vi "_UserDialog Choose ReadMe Params.vi"(0 "VI Default Path":path, 1 "LV <help> directory?":bool, 2 "Documentable VI Path":path, 7 "Info extracted from old HTML":T1={"_vi_name_"="", "_vi_description_text_"="", "_vi_controls_and_indicators_descriptions_"="", "_name_of_owning_library_"="", "_owning_library_html_"="", "_Packages_"="Base Package", "_Platforms_"="Windows", "_details_text_"="Put details here", "_example_screenshot_"="", "_example_vi_"="", "_path_to_example_file_"=path "", "IsDetailsON?"=FALSE, "IsOwningLibraryON?"=FALSE, "IsExamplesON?"=FALSE, "IsTableON?"=FALSE, "IsScrollableON?"=FALSE, "IsDetailedHelpLinkON?"=FALSE, "Table Objects array"=[], "Table Descriptions array"=[], "Table Links array"=[], "Start path location"=enum."VI folder"}, 11 "error in (no error)":errorcluster) -> (4 "HTML File Path":path, 8 "VI Info":T1={"_vi_name_"="", "_vi_description_text_"="", "_vi_controls_and_indicators_descriptions_"="", "_name_of_owning_library_"="", "_owning_library_html_"="", "_Packages_"="Base Package", "_Platforms_"="Windows", "_details_text_"="Put details here", "_example_screenshot_"="", "_example_vi_"="", "_path_to_example_file_"=path "", "IsDetailsON?"=FALSE, "IsOwningLibraryON?"=FALSE, "IsExamplesON?"=FALSE, "IsTableON?"=FALSE, "IsScrollableON?"=FALSE, "IsDetailedHelpLinkON?"=FALSE, "Table Objects array"=[], "Table Descriptions array"=[], "Table Links array"=[], "Start path location"=enum."VI folder"}, 14 "Cancelled by User?":bool, 15 "error out":errorcluster)   [LabVIEW 2012]
uses:
  _Controls and TypeDefs/UserDialogStates.ctl
  _Controls and TypeDefs/InfoFromOldHTML_cluster.ctl
  _Controls and TypeDefs/StartPathLocation_enum.ctl
  <vilib>/Platform/browser.llb/Open URL in Default Browser (string).vi
panel:
  in  "www.labicom.net":bool
  in  "Help Button":bool
  in  "Disclaimer":string="[Disclaimer text]"
  in  "IsDisclaimer? chkBox":bool=TRUE
  in  "Cancel Button":bool
  in  "GenerateReadme_btn":bool
  in  "Patents":string="[Patents text]"
  in  "Trademarks":string="[Trademarks text]"
  in  "Copyright":string="[Copyright text]"
  in  "Support CommunityForums":string=" [link to community forums or NI Community page and expected response time]"
  in  "SupportEmail":string="[Support email address and expected response time]"
  in  "SupportTelephone":string="[Telephone number and hours of operation]"
  in  "AppUpgrader":string="[Developer Name, Developer e-mail, Developer certification level (if any), Organization]"
  out "Product Version 8":string="[Version#]" caption="Product Version"
  in  "AppDeveloper":string="[Developer Name, Developer e-mail, Developer certification level (if any), Organization]"
  out "Product Short Name 12":string="[ProductShortName]" caption="Product Short Name"
  in  "IsDeveloper? chkBox":bool=TRUE
  in  "FixedIssues Table":string[][](table)=[["[#]", "[Summary Text]"], ["", ""], ["", ""]]
  out "Product Version 7":string="[Version#]" caption="Product Version"
  out "Product Short Name 11":string="[ProductShortName]" caption="Product Short Name"
  in  "NewFeatures Table":string[][](table)=[["[Feature 1]"], ["[Feature 2]"], [""]]
  out "Product Version 6":string="[Version#]" caption="Product Version"
  out "Product Short Name 10":string="[ProductShortName]" caption="Product Short Name"
  out "Product Version 5":string="[Version#]" caption="Product Version"
  out "Product Short Name 9":string="[ProductShortName]" caption="Product Short Name"
  in  "UpgradeIssuesDescription":string="[Description of known upgrade issue included recommended workaround.]"
  in  "Upgrade Issue Heading":string="[Upgrade Issue Heading]"
  out "Product Short Name 8":string="[ProductShortName]" caption="Product Short Name"
  in  "Device Support Table":string[][](table)=[["[Device]"], ["[Device]"], [""]]
  out "Product Short Name 7":string="[ProductShortName]" caption="Product Short Name"
  out "Product Short Name 6":string="[ProductShortName]" caption="Product Short Name"
  in  "NI Software Support Table":string[][](table)=[["LabVIEW", "8.5.x, 8.6.x, 2009 and later"], ["LabVIEW Real-Time Module", "8.5.x and later (including 2009 and later)"]]
  out "Product Version 4":string="[Version#]" caption="Product Version"
  out "Product Short Name 5":string="[ProductShortName]" caption="Product Short Name"
  in  "Additional OS remarks":string="[ProductName] [Version#] supports Phar Lap only with the LabVIEW Real-Time Module 8.5 and later.\nTo find and download an earlier version of [ProductName] [Version#] that supports other operating systems, refer to [link to older versions]."
  in  "Caution Text":string
  in  "OS Note":string="[Support for Windows Server 2003 R2 may require ...]"
  in  "OperatingSystems Table":string[][](table)=[["Windows 7 (32-bit and 64-bit)"], [""], [""], [""], [""]]
  out "Product Version 3":string="[Version#]" caption="Product Version"
  out "Product Short Name 4":string="[ProductShortName]" caption="Product Short Name"
  out "Product Short Name 3":string="[ProductShortName]" caption="Product Short Name"
  in  "SystemRequirements Table":string[][](table)=[["Development", "1 GB", "1 GHz or better"], ["Deployment", "256 MB", "600 MHz or better"]]
  in  "Installation Instructions":string[][](table)=[["[Step 1]"], ["[Step 2]"], [""], [""]]
  out "Product Short Name 2":string="[ProductShortName]" caption="Product Short Name"
  in  "IsCopyright? chkBox":bool=TRUE
  in  "IsPatents? chkBox":bool=TRUE
  in  "IsFixedIssues? chkBox":bool=TRUE
  in  "IsDeviceSupport? chkBox":bool=TRUE
  in  "IsTrademarks? chkBox":bool=TRUE
  in  "IsContactSupport? chkBox":bool=TRUE
  in  "IsNewFeatures? chkBox":bool=TRUE
  in  "IsUpgradeIssues? chkBox":bool=TRUE
  in  "IsSoftwareSupport? chkBox":bool=TRUE
  in  "IsSysRequirements? chkBox":bool=TRUE
  in  "IsInstallation? chkBox":bool=TRUE
  out "Product Version 2":string="[Version#]" caption="Product Version"
  in  "Product Short Name":string="[ProductShortName]"
  in  "Year":string="[Year]"
  in  "Month":string="[Month]"
  in  "Product Version":string="[Version#]"
  in  "Product Full Name":string="[ProductFullName]"
  in  "Next_btn":bool
  in  "UserDialogSteps":T3=enum."Choose parameters"
  # "Readme"
  # "Thank you for using"
  # ", version"
  # "."
  # "The readme contains the following main sections:"
  # "Installation (if applicable)"
  # "."
  # "This section documents installation instructions for"
  # "New line here corresponds to new item in the list in HTML"
  # "System Requirements (if applicable)"
  # "Software Support in"
  # "(if applicable)"
  # "Operating System Support"
  # ":"
  # "The following operating systems are supported in"
  # "Step 2/2:\nConfigure VI Documentation Layout"
  # "Note"
  # "Additional layout elements for LabVIEW help"
  # "This icon denotes a note, which alerts you\nto important information. You can add it\nby placing <_note_> into your text."
  # "Caution: place <_caution_> into your text"
  # "Caution"
  # "Note: place <_note_> into your text"
  # "This icon denotes a caution, which \nadvises you of precautions to take to \navoid injury, data loss, or a system crash.\nYou can add it by placing <_caution_>\ninto your text."
  # "Mandatory Fields"
  # "Tip: place <_tip_> into your text"
  # "Windows"
  # "Platform: enclose platform name between\n<_platform_> and </_platform_> tags"
  # "Text in blue color denotes a specific \nplatform and indicates that the text \nfollowing it applies only to that platform.\nYou can add it enclosing platform name\nbetween <_platform_> and </_platform_>\ntags (e.g.: <_platform_>MacOS X</_platform_>)."
  # "NI Application Software Support"
  # "The following table lists the NI application software versions supported by"
  # "bold"
  # "Text in bold: enclose such text between\n<B> and </B> tags"
  # ":"
  # "Attention!"
  # "Caution Text: enclose such text between \n<_caution_text_> and </_caution_text_> tags"
  # "Bold text denotes items that you must \nselect or click on in the software, such as \nmenu items and dialog box options. \nBold text also denotes parameter names, \nemphasis, or an introduction to a key \nconcept. You can emphasize such text by \nenclosing in between <B> and </B> tags."
  # "vigods.com"
  # "Link: place relative path in place of '_path_' and\ntext in place of '_text_' and insert resulting string\nwherever you need: \n<a href=\"_path_\">_text_</a>"
  # "monospace"
  # "Monospace: enclose such text between\n<_monospace_> and </_monospace_> tags"
  # "Device Support in"
  # "(if applicable)"
  # "The following lists detail the devices supported in"
  # "."
  # "Upgrade and Compatibility Issues"
  # "(if applicable)"
  # "This section covers changes in"
  # "functionality."
  # "New Features Added in"
  # "(if applicable)"
  # ":"
  # "The following features were added in"
  # "Fixed Issues"
  # "(if applicable)"
  # "The following issues were fixed in"
  # "Developer(s) of"
  # "(if applicable)"
  # "This application was developed by"
  # "Last upgrade of this application (to the version"
  # ") was made by"
  # "Contact Support"
  # "(if applicable)"
  # "You can contact our support staff by one of the following:"
  # "Telephone:"
  # "Email:"
  # "Community Forums:"
  # "Copyright"
  # "(if applicable)"
  # "Trademarks"
  # "(if applicable)"
  # "Patents"
  # "(if applicable)"
  # "Disclaimer"
  # "(if applicable)"
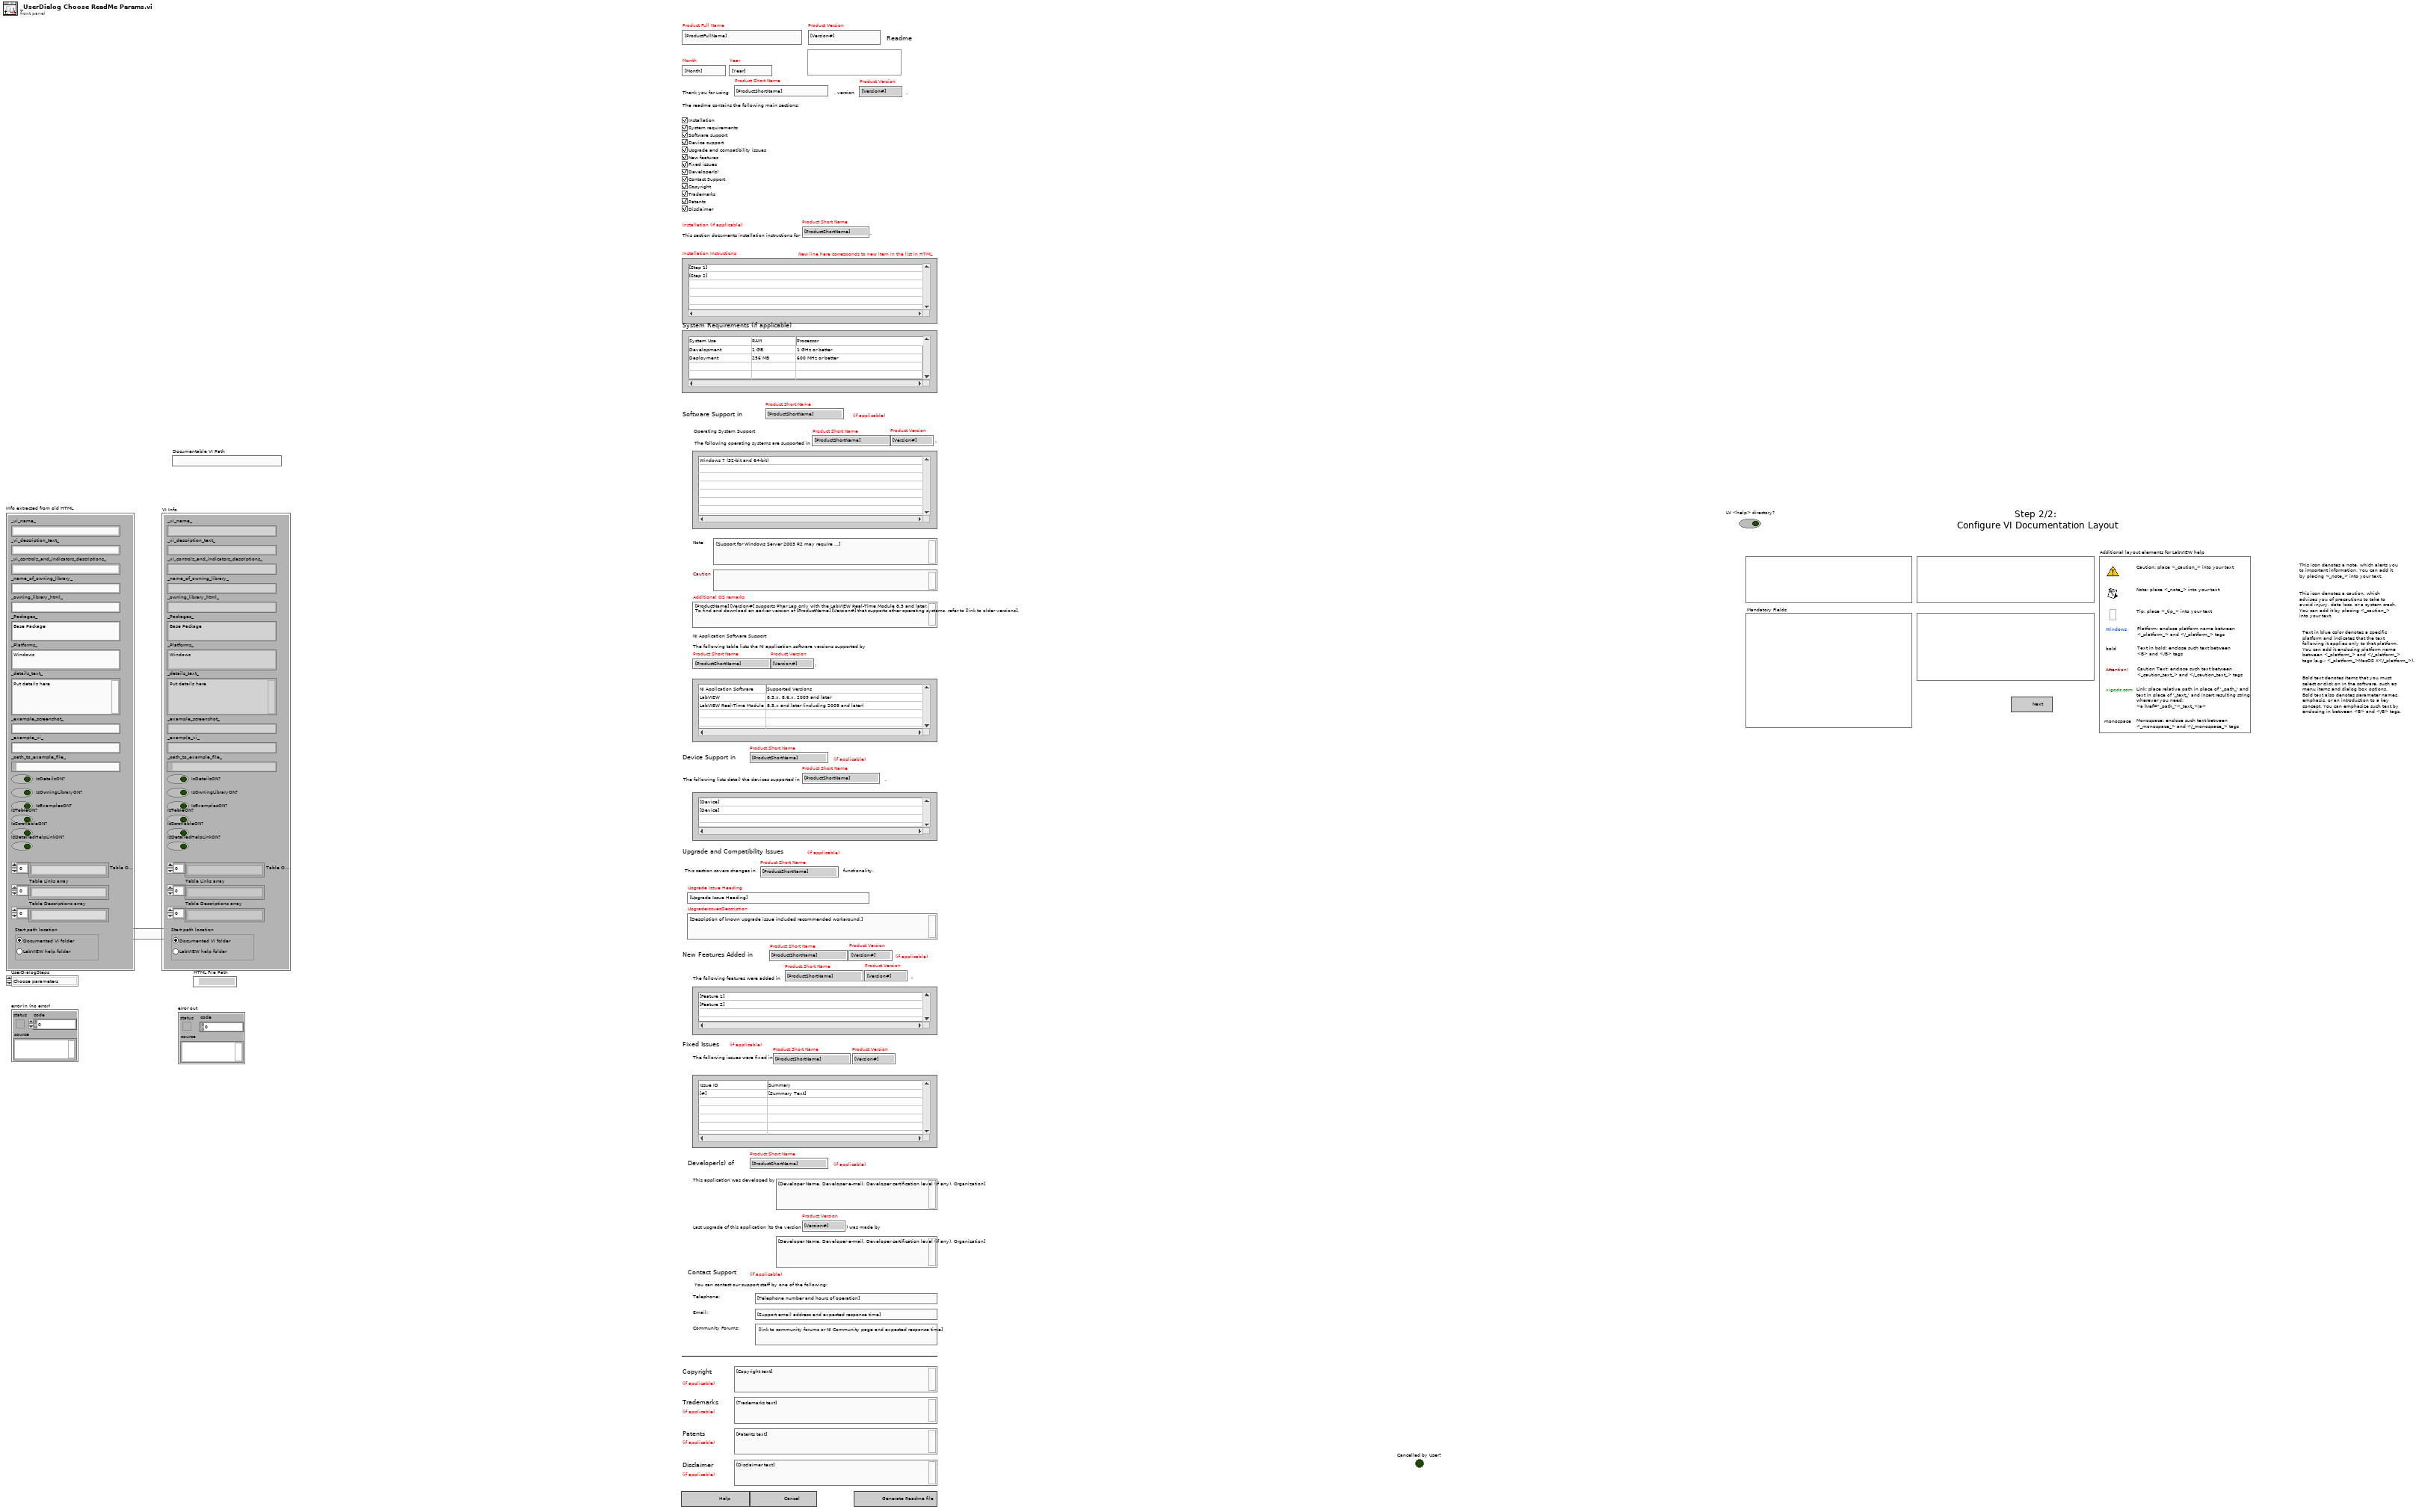
[diagram p1: front panel]
types:
  T1 = typedef "InfoFromOldHTML_cluster.ctl" = cluster{"_vi_name_":string, "_vi_description_text_":string, "_vi_controls_and_indicators_descriptions_":string, "_name_of_owning_library_":string, "_owning_library_html_":string, "_Packages_":string, "_Platforms_":string, "_details_text_":string, "_example_screenshot_":string, "_example_vi_":string, "_path_to_example_file_":path, "IsDetailsON?":bool, "IsOwningLibraryON?":bool, "IsExamplesON?":bool, "IsTableON?":bool, "IsScrollableON?":bool, "IsDetailedHelpLinkON?":bool, "Table Objects array":string[], "Table Descriptions array":string[], "Table Links array":string[], "Start path location":T2}
  T2 = typedef "StartPathLocation_enum.ctl" = enum32{"VI folder", "Help folder"}
  T3 = typedef "UserDialogStates.ctl" = enum16{"Overview", "Known Issues", "Choose parameters", "Update", "Choose HTML file path", "Choose Images directory path", "Decide if there is Context Help", "Choose help hierarchy", "Generate HTML", "Installation", "System Requirements", "Software Support", "Device Support", "Upgrade Issues", "New Features", "Fixed Issues", "Developer", "Contact Support", "Copyright", "Trademarks", "Patents", "Disclaimer", "Save", "Shutdown"}
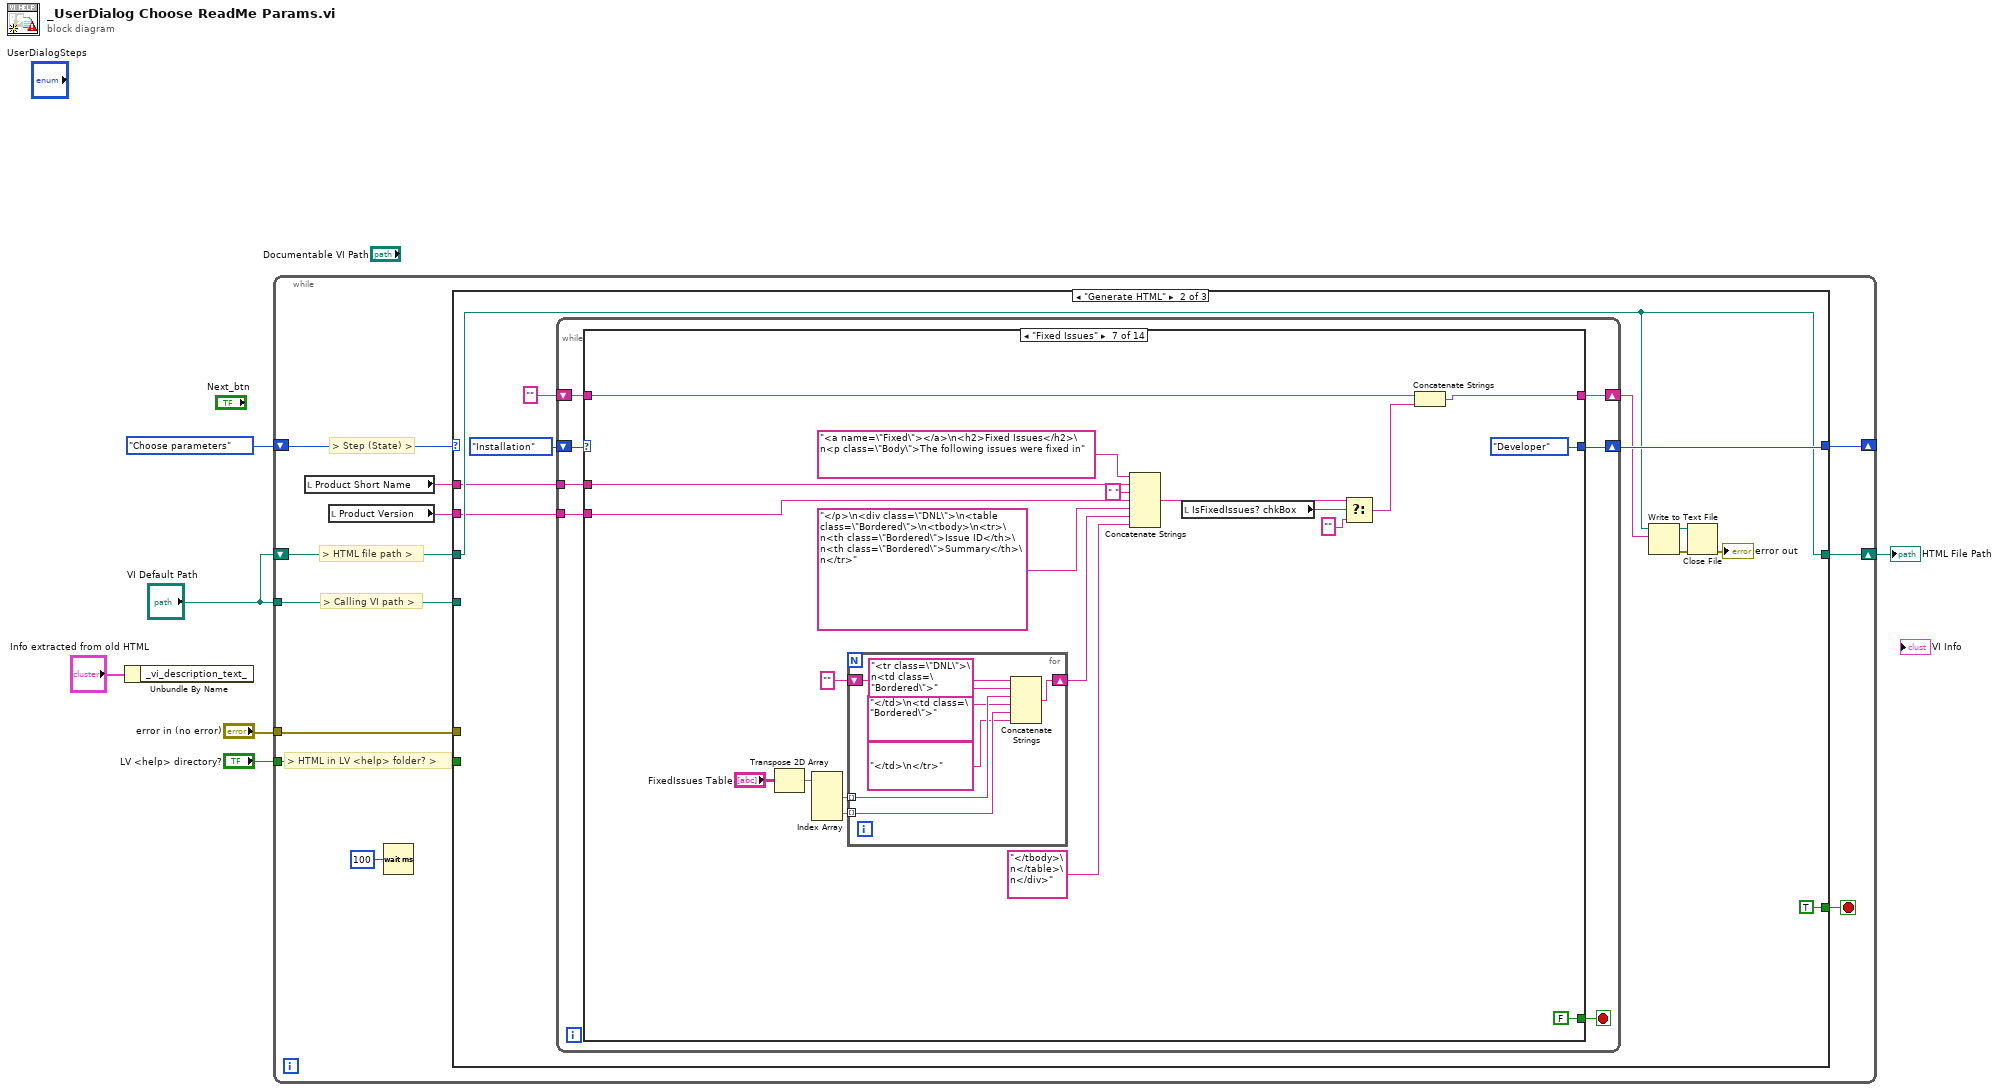
[diagram p0: block diagram]
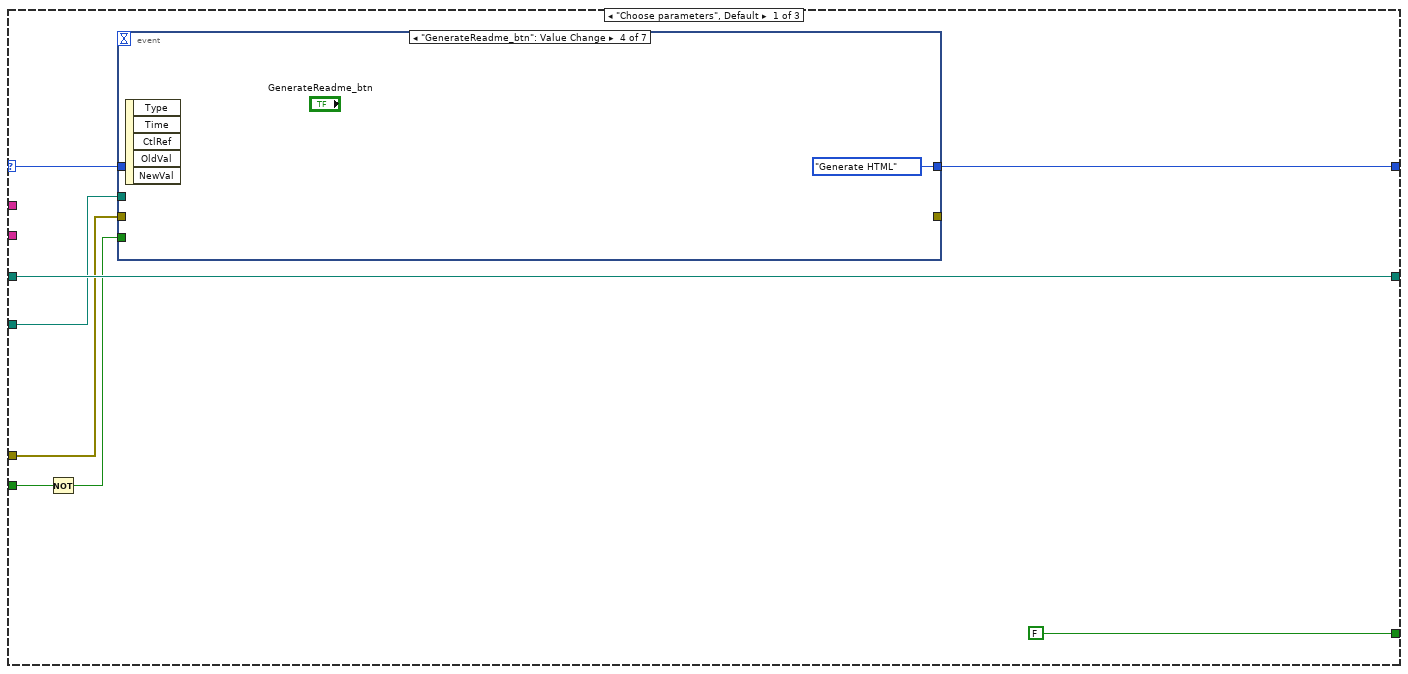
[diagram p2: hidden frame]
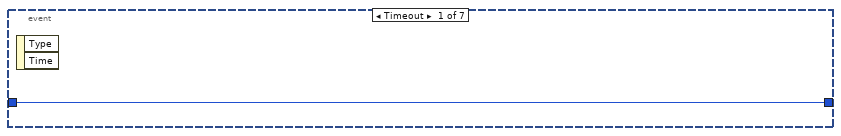
[diagram p3: hidden frame]
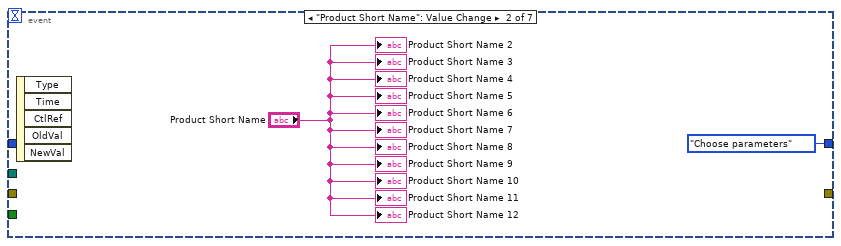
[diagram p4: hidden frame]
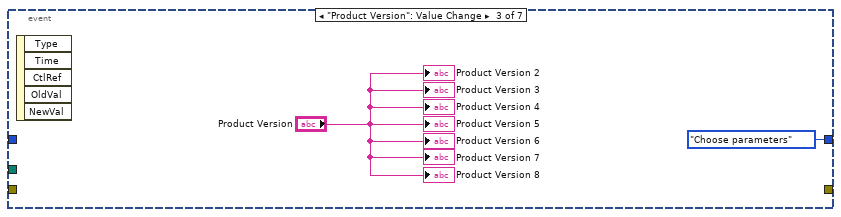
[diagram p5: hidden frame]
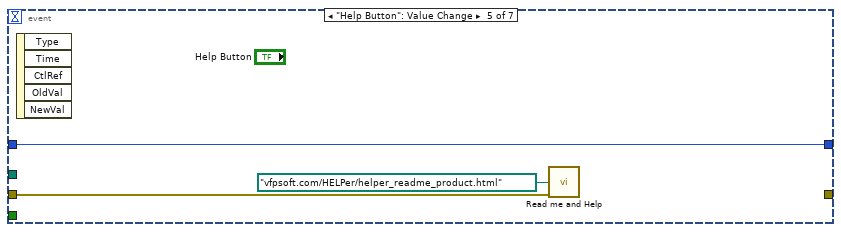
[diagram p6: hidden frame]
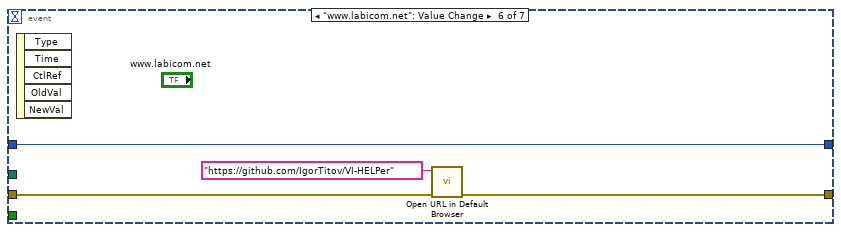
[diagram p7: hidden frame]
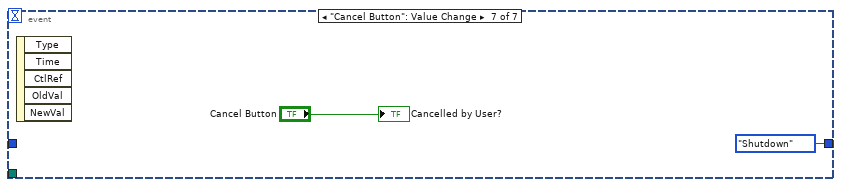
[diagram p8: hidden frame]
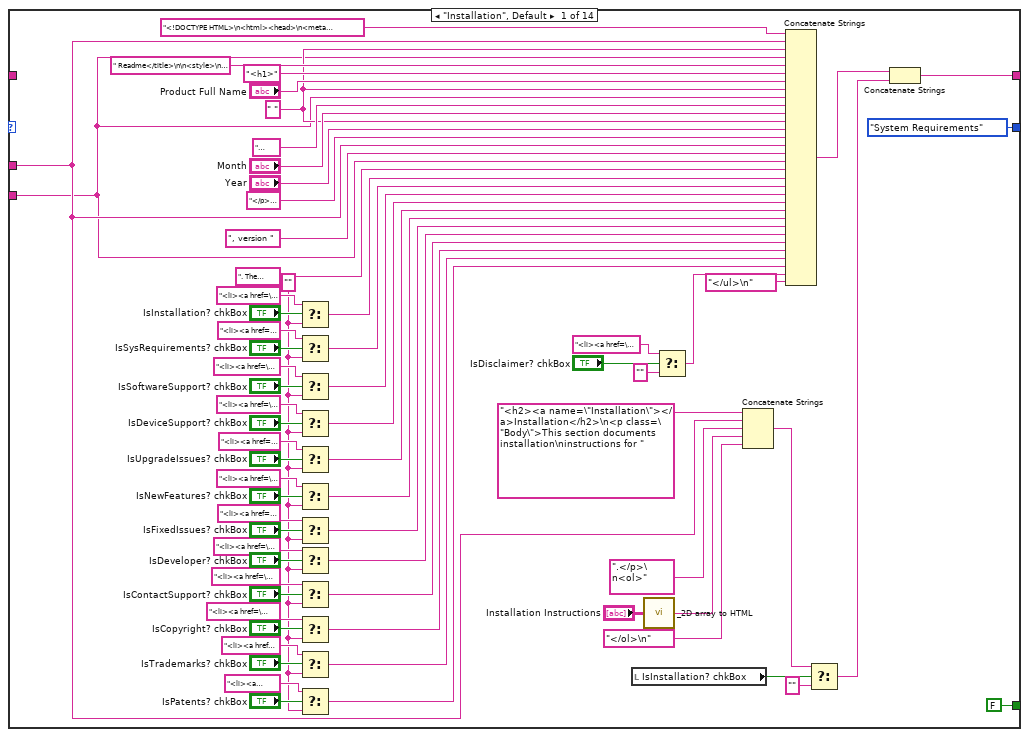
[diagram p9: hidden frame]
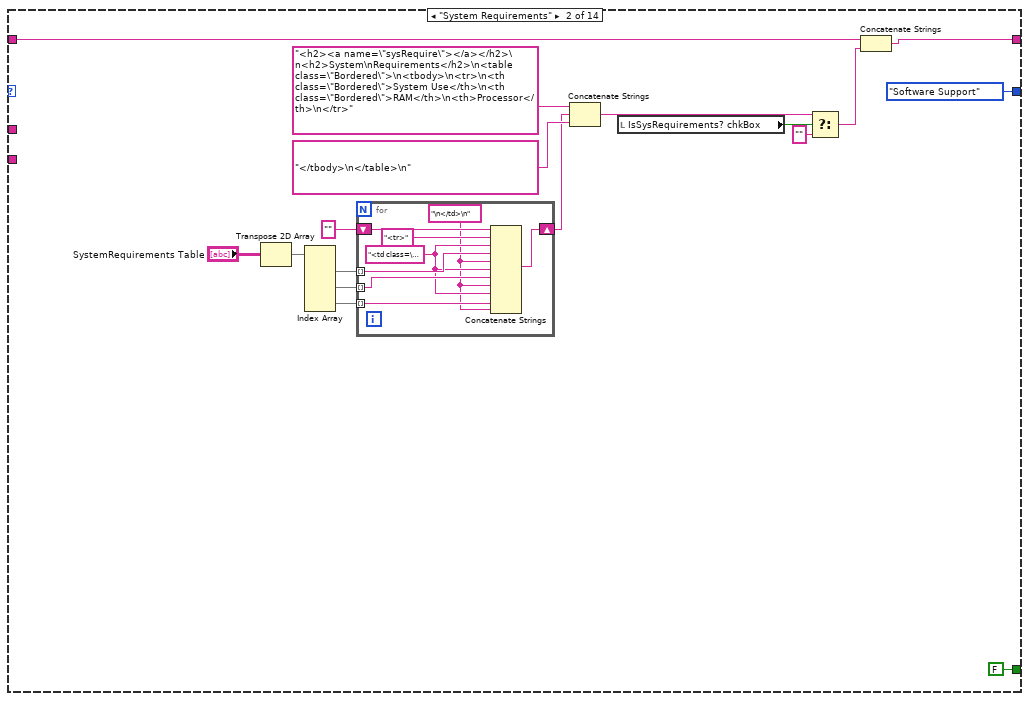
[diagram p10: hidden frame]
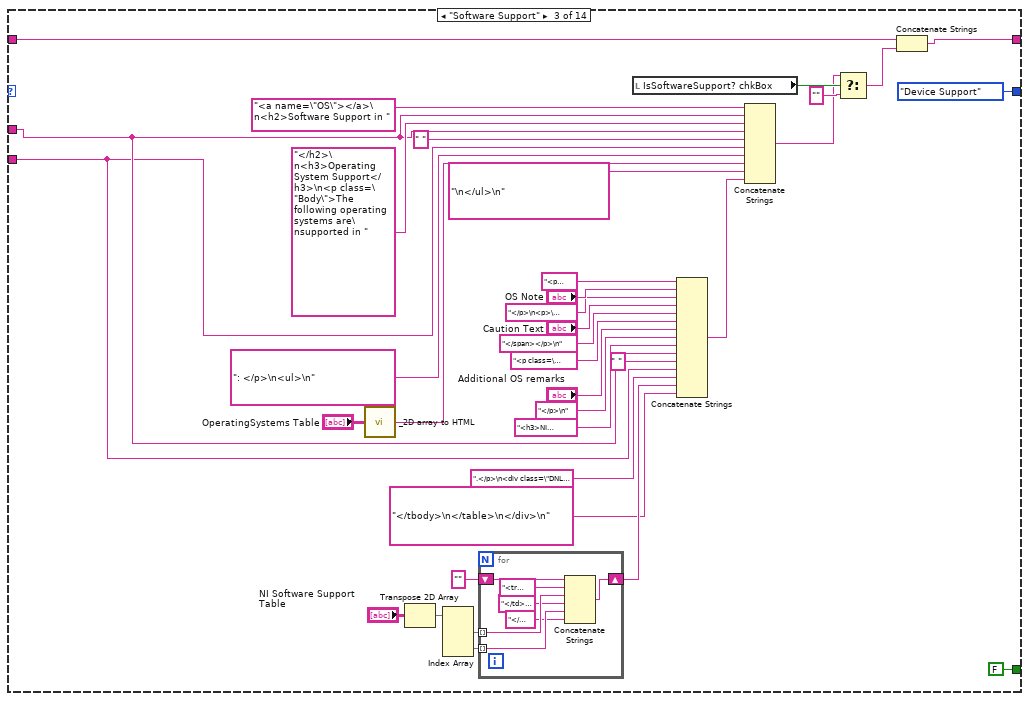
[diagram p11: hidden frame]
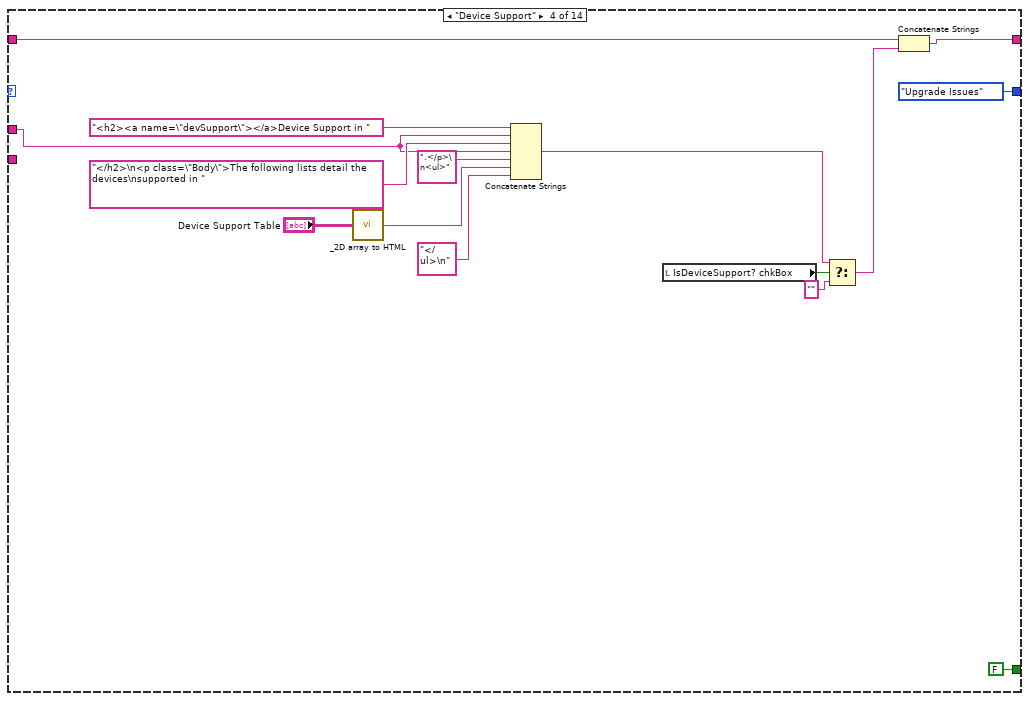
[diagram p12: hidden frame]
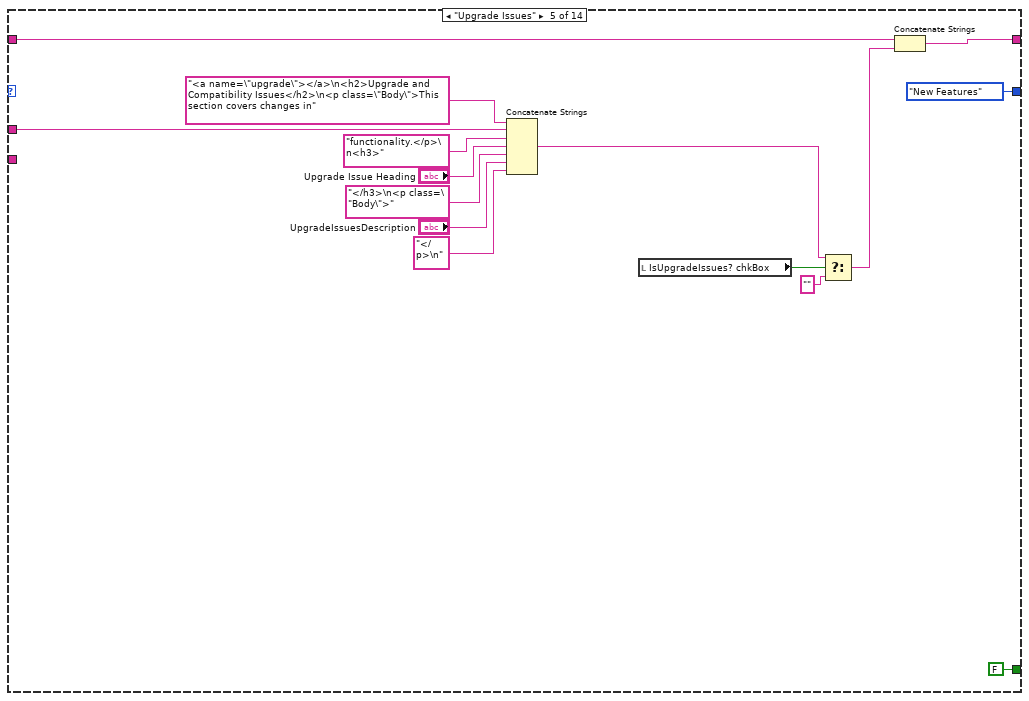
[diagram p13: hidden frame]
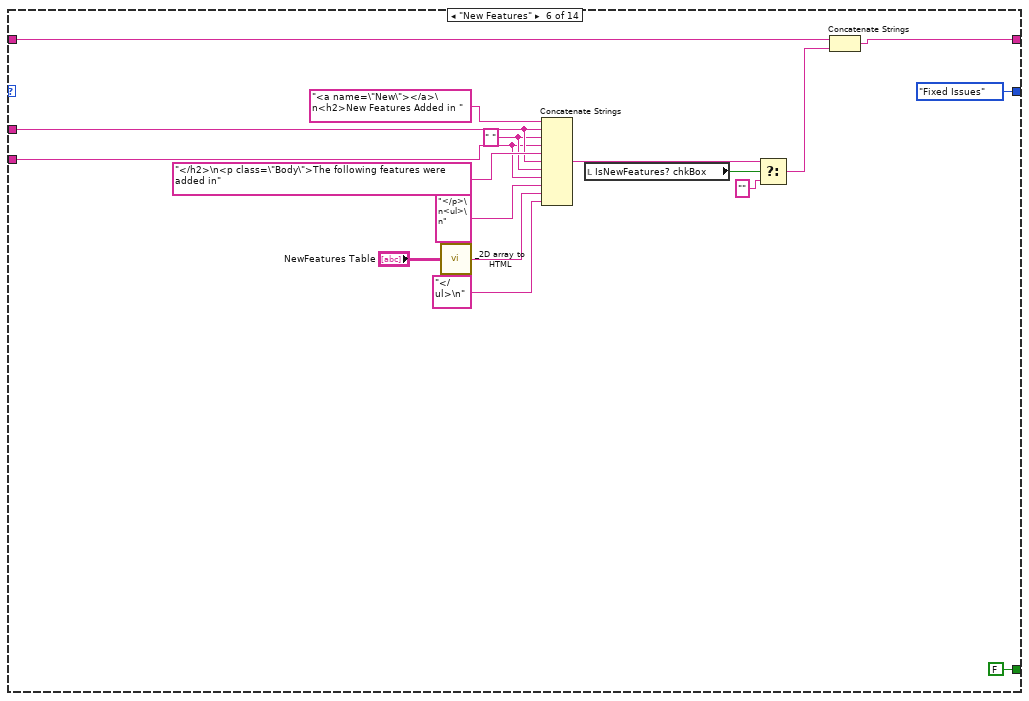
[diagram p14: hidden frame]
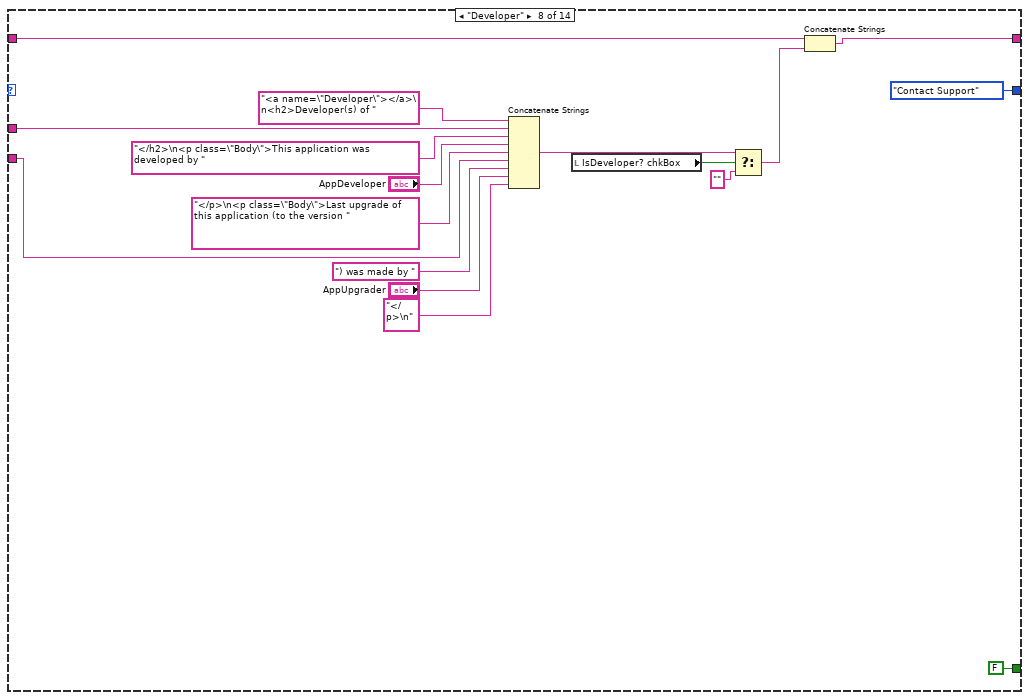
[diagram p15: hidden frame]
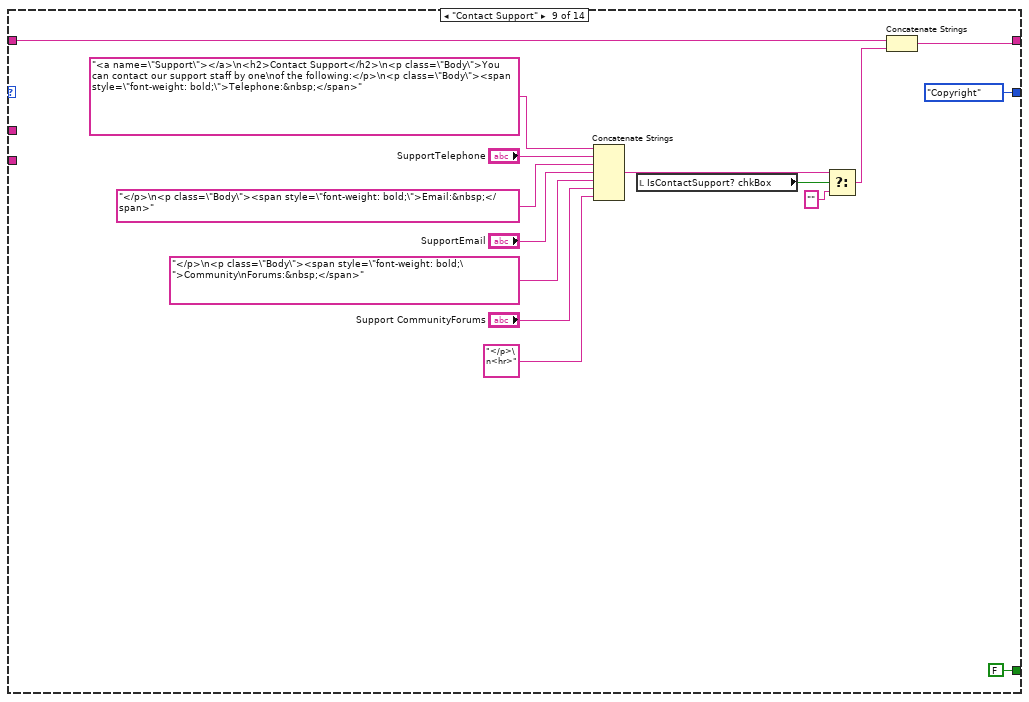
[diagram p16: hidden frame]
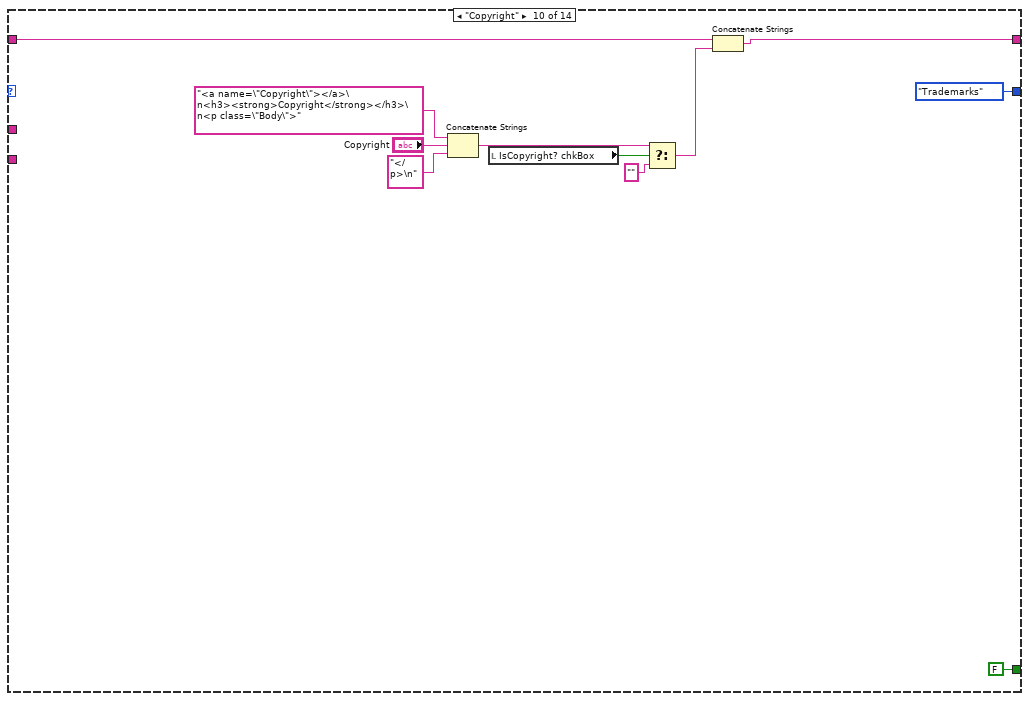
[diagram p17: hidden frame]
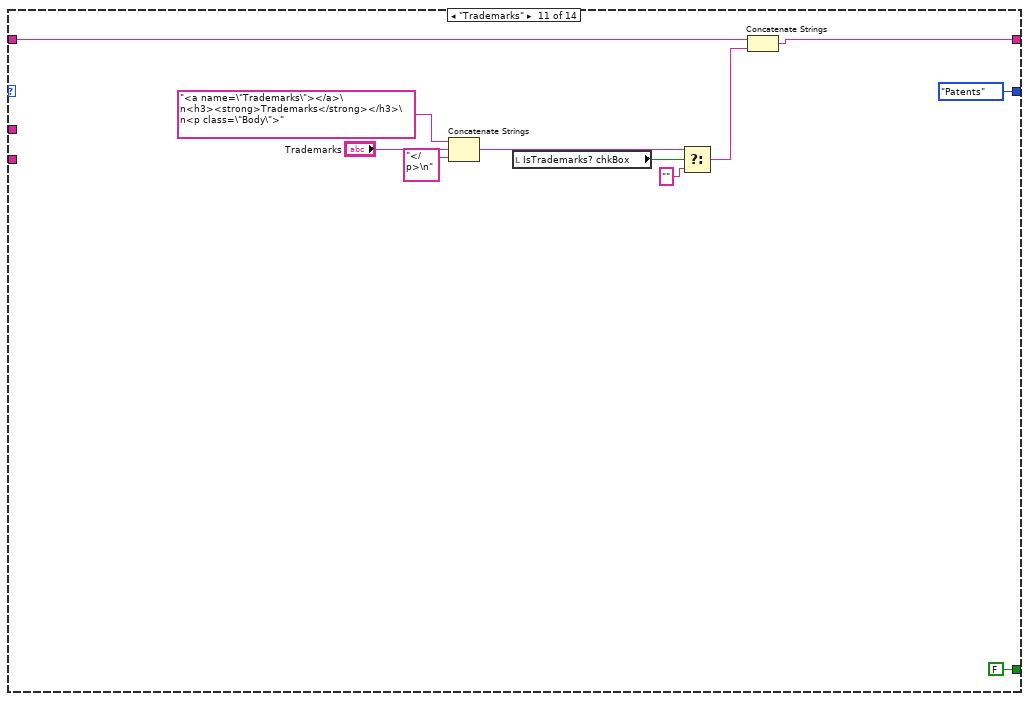
[diagram p18: hidden frame]
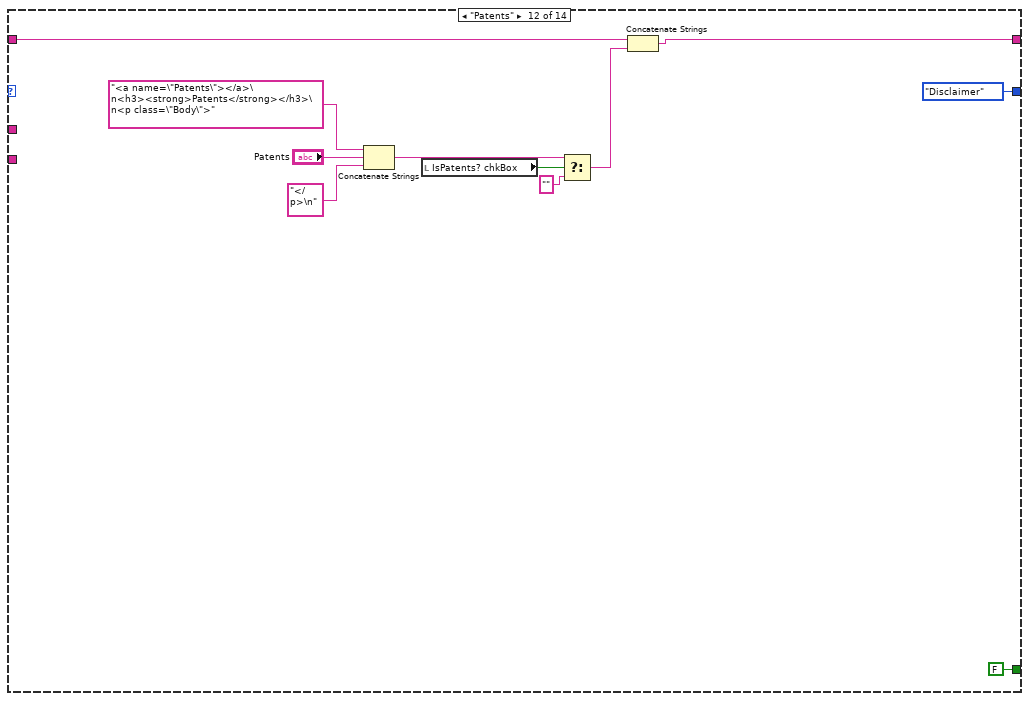
[diagram p19: hidden frame]
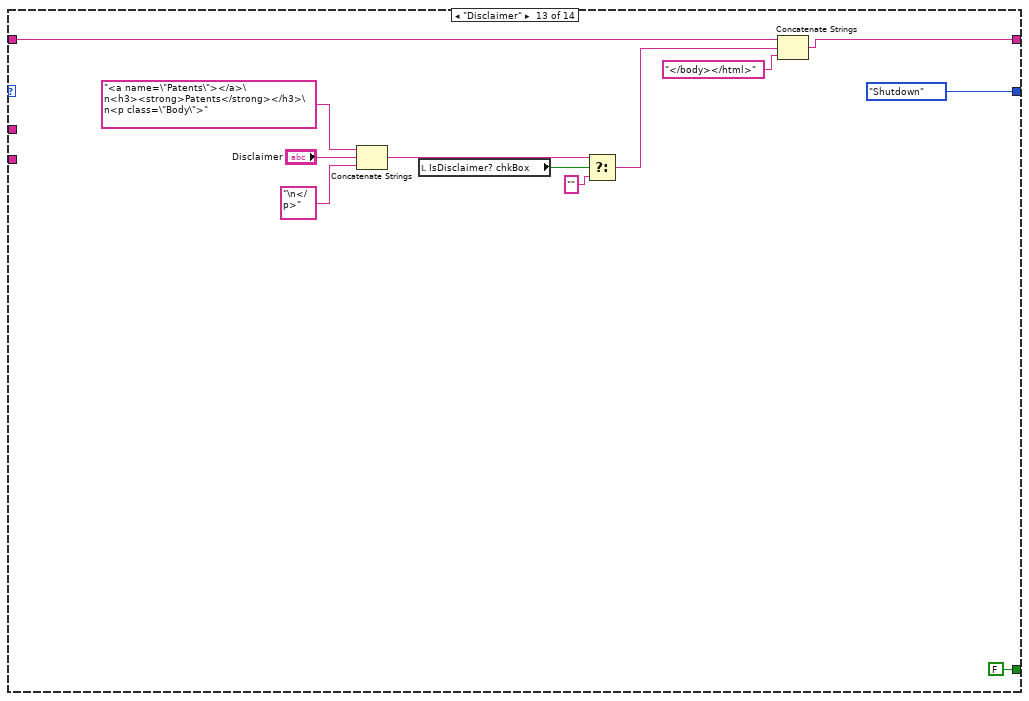
[diagram p20: hidden frame]
diagram:
  n1 = Unbundle By Name("Info extracted from old HTML") -> ()  [unwired: 1 out]
  n2 = while {
    shift-right: [w14] -> _
    shift-left: UserDialogStates."Choose parameters" ("UserDialogSteps") -> [w15]
    tunnel: "VI Default Path" -> [w13]
    shift-right: [w12] -> w3
    shift-left: "VI Default Path" -> [w11]
    tunnel: "LV <help> directory?" -> [w10]
    tunnel: "error in (no error)" -> [w9]
    stop <- w17 stop-if-true
    # "> HTML in LV <help> folder? >"
    # "> Step (State) >"
    # "> Calling VI path >"
    # "> HTML file path >"
    n3 = local read "Product Short Name"() -> (w8:string)
    n4 = local read "Product Version"() -> (w7:string)
    n5 = Wait (ms)(milliseconds to wait=u32 100) -> ()  [unwired: 1 out]
    n6 = case shown="\"Generate HTML\"" w15 {
      selector: w15 -> [w24 _ _]
      tunnel: [FALSE TRUE TRUE] -> w17
      tunnel: [w23 w49 UserDialogStates."Shutdown" ("UserDialogSteps")] -> w14
      tunnel: w13 -> [w20 _ _]
      tunnel: [w22 w47 w350] -> w12
      tunnel: w11 -> [w22 w47 w350]
      tunnel: w10 -> [w21 _ _]
      tunnel: w9 -> [w18 _ _]
      tunnel: w8 -> [_ w42 _]
      tunnel: w7 -> [_ w41 _]
      frame "Choose parameters", Default {
        n7 = Not(x=w21) -> (.not. x?=w19:bool)
        n8 = event shown="[3] \"GenerateReadme_btn\": Value Change" {
          selector: _ -> [_ _ _ _ _ _ _]
          dyn-events: _ -> [_ _ _ _ _ _ _]
          timeout: _ -> [_ _ _ _ _ _ _]
          tunnel: w24 -> [w26 _ _ _ w32 w38 _]
          tunnel: [w26 UserDialogStates."Choose parameters" ("UserDialogSteps") UserDialogStates."Choose parameters" ("UserDialogSteps") UserDialogStates."Generate HTML" ("UserDialogSteps") w32 w38 UserDialogStates."Shutdown" ("UserDialogSteps")] -> w23
          tunnel: w20 -> [_ _ _ _ _ _ _]
          tunnel: w19 -> [_ _ _ _ _ _ _]
          tunnel: w18 -> [_ _ _ _ w33 w36 _]
          tunnel: [_ _ _ _ _ w35 _] -> _
          event Timeout {
            n9 = event-data() -> ()  [unwired: 1 in, 2 out]
          }
          event "Product Short Name": Value Change {
            n10 = event-data() -> ()  [unwired: 1 in, 5 out]
            "Product Short Name 2" <- "Product Short Name"
            "Product Short Name 9" <- "Product Short Name"
            "Product Short Name 3" <- "Product Short Name"
            "Product Short Name 4" <- "Product Short Name"
            "Product Short Name 5" <- "Product Short Name"
            "Product Short Name 6" <- "Product Short Name"
            "Product Short Name 7" <- "Product Short Name"
            "Product Short Name 8" <- "Product Short Name"
            "Product Short Name 10" <- "Product Short Name"
            "Product Short Name 11" <- "Product Short Name"
            "Product Short Name 12" <- "Product Short Name"
          }
          event "Product Version": Value Change {
            n11 = event-data() -> ()  [unwired: 1 in, 5 out]
            "Product Version 2" <- "Product Version"
            "Product Version 3" <- "Product Version"
            "Product Version 4" <- "Product Version"
            "Product Version 5" <- "Product Version"
            "Product Version 6" <- "Product Version"
            "Product Version 7" <- "Product Version"
            "Product Version 8" <- "Product Version"
          }
          event "GenerateReadme_btn": Value Change {
            n12 = event-data() -> ()  [unwired: 1 in, 5 out]
          }
          event "Help Button": Value Change {
            n13 = event-data() -> ()  [unwired: 1 in, 5 out]
            n14 = call "Read me and Help.vi"("path"=path "vfpsoft.com/HELPer/helper_readme_product.html", "error in"=w33) -> ()  [unwired: 13 in, 1 out]
          }
          event "www.labicom.net": Value Change {
            n15 = event-data() -> ()  [unwired: 1 in, 5 out]
            n16 = call-poly <vilib>:"Open URL in Default Browser.vi"("error in (no error)"=w36, "URL"="https://github.com/IgorTitov/VI-HELPer") -> ("error out"=w35:errorcluster)  [unwired: 4 in, 1 out]
          }
          event "Cancel Button": Value Change {
            n17 = event-data() -> ()  [unwired: 1 in, 5 out]
            "Cancelled by User?" <- "Cancel Button"
          }
        }
      }
      frame "Generate HTML" {
        n18 = while {
          shift-right: [w57] -> w49
          shift-left: UserDialogStates."Installation" ("UserDialogSteps") -> [w58]
          shift-right: [w55] -> w46
          shift-left: "" -> [w56]
          tunnel: w42 -> [w53]
          tunnel: w41 -> [w52]
          stop <- w54 stop-if-true
          n19 = case shown="\"Fixed Issues\"" w58 {
            tunnel: [UserDialogStates."System Requirements" ("UserDialogSteps") UserDialogStates."Software Support" ("UserDialogSteps") UserDialogStates."Device Support" ("UserDialogSteps") UserDialogStates."Upgrade Issues" ("UserDialogSteps") UserDialogStates."New Features" ("UserDialogSteps") UserDialogStates."Fixed Issues" ("UserDialogSteps") UserDialogStates."Developer" ("UserDialogSteps") UserDialogStates."Contact Support" ("UserDialogSteps") UserDialogStates."Copyright" ("UserDialogSteps") UserDialogStates."Trademarks" ("UserDialogSteps") UserDialogStates."Patents" ("UserDialogSteps") UserDialogStates."Disclaimer" ("UserDialogSteps") UserDialogStates."Shutdown" ("UserDialogSteps") UserDialogStates."Shutdown" ("UserDialogSteps")] -> w57
            tunnel: w56 -> [_ w142 w176 w207 w219 w237 w257 w282 w296 w307 w318 w329 w340 w346]
            tunnel: [w80 w141 w175 w206 w220 w238 w256 w281 w295 w306 w317 w328 w343 w346] -> w55
            tunnel: [FALSE FALSE FALSE FALSE FALSE FALSE FALSE FALSE FALSE FALSE FALSE FALSE FALSE TRUE] -> w54
            tunnel: w53 -> [w60 _ w153 w195 w215 w234 w252 w276 _ _ _ _ _ _]
            tunnel: w52 -> [w59 _ w152 _ _ w232 w250 w272 _ _ _ _ _ _]
            frame "Installation", Default {
              w83 = ""
              w61 = " " ("string")
              n20 = Select(t="<li><a href=\"#Installation\">Installation</a></li>\n", s="IsInstallation? chkBox", f=w83) -> (s? t:f=w116:string)
              n21 = Select(t="<li><a href=\"#sysRequire\">System requirements</a></li>\n", s="IsSysRequirements? chkBox", f=w83) -> (s? t:f=w113:string)
              n22 = Select(t="<li><a href=\"#OS\">Software support</a></li>\n", s="IsSoftwareSupport? chkBox", f=w83) -> (s? t:f=w110:string)
              n23 = Select(t="<li><a href=\"#devSupport\">Device support</a></li>\n", s="IsDeviceSupport? chkBox", f=w83) -> (s? t:f=w108:string)
              n24 = Select(t="<li><a href=\"#upgrade\">Upgrade and compatibility issues</a></li>\n", s="IsUpgradeIssues? chkBox", f=w83) -> (s? t:f=w104:string)
              n25 = Select(t="<li><a href=\"#New\">New features</a></li>\n", s="IsNewFeatures? chkBox", f=w83) -> (s? t:f=w102:string)
              n26 = Select(t="<li><a href=\"#Fixed\">Fixed issues</a></li>\n", s="IsFixedIssues? chkBox", f=w83) -> (s? t:f=w99:string)
              n27 = Select(t="<li><a href=\"#Developer\">Developer(s)</a></li>", s="IsDeveloper? chkBox", f=w83) -> (s? t:f=w96:string)
              n28 = Select(t="<li><a href=\"#Support\">Contact Support</a></li>\n", s="IsContactSupport? chkBox", f=w83) -> (s? t:f=w93:string)
              n29 = Select(t="<li><a href=\"#Copyright\">Copyright</a></li>\n", s="IsCopyright? chkBox", f=w83) -> (s? t:f=w89:string)
              n30 = Select(t="<li><a href=\"#Trademarks\">Trademarks</a></li>\n", s="IsTrademarks? chkBox", f=w83) -> (s? t:f=w82:string)
              n31 = Select(t="<li><a href=\"#Patents\">Patents</a></li>\n", s="IsPatents? chkBox", f=w83) -> (s? t:f=w81:string)
              n32 = local read "IsInstallation? chkBox"() -> (w77:bool)
              n33 = call "_2D array to HTML.vi"("Table (2D Array)"="Installation Instructions") -> ("HTML Code"=w73:string)  [unwired: 14 in]
              n34 = Select(t="<li><a href=\"#Disclaimer\">Disclaimer</a></li>\n", s="IsDisclaimer? chkBox", f="") -> (s? t:f=w67:string)
              n35 = Concatenate Strings("<h2><a name=\"Installation\"></a>Installation</h2>\n<p class=\"Body\">This section documents installation\ninstructions for " ("string"), w60, ".</p>\n<ol>" ("string"), w73, "</ol>\n" ("string")) -> (w71:string)
              n36 = Concatenate Strings("<!DOCTYPE HTML>\n<html><head>\n<meta http-equiv=\"Content-Type\" content=\"text/html; charset=ISO-8859-1\">\n<META NAME=\"GENERATOR\" CONTENT=\"HELPer - VI Documentation Toolkit from https://github.com/IgorTitov/VI-HELPer\">\n<script>\nfunction Link(URL)\n{\nwindow.location = URL;\n}\n</script>\n<meta http-equiv=\"Content-Type\" content=\"text/html; charset=ISO-8859-1\"><title>", w60, w61, w59, " Readme</title>\n\n<style>\n/***************************************************/\n/* MINIMAL STYLES */\n/* The following section defines styles that every HTML Help project should\nneed. */\n/* The default style of P is red to alert you that you need to apply a style\nclass, such as Body. */\nP { margin-top:6.00pt; margin-bottom:6.00pt; font-family:Verdana; font-size:8pt;\ncolor: #FF0000; }\nBR { font-size:4.00pt; }\n/* Use H1 for all topic headings. */\nH1 { margin-top:3.00pt; margin-bottom:3.00pt; font-family:Verdana;\nfont-size:12pt; font-weight:bold; }\n/* Use H2 for second-level headings. */\nH2 { margin-top:9.00pt; margin-bottom:3.00pt; font-family:Verdana;\nfont-size:10pt; font-weight:bold; }\n/* Use H3 for third-level headings. */\nH3 { margin-top:6.00pt; margin-bottom:3.00pt; font-family:Verdana;\nfont-size:8pt; font-weight:bold; }\n/* Use H4 for fourth-level headings. */\nH4 { margin-top:3.00pt; margin-bottom:3.00pt; font-family:Verdana;\nfont-size:8pt; font-weight:bold; }\n/* H5 and H6 have the same definition as H4 because you should not need this\nlevel of heading in one topic. If you need to use H5 or H6, consider breaking up\nyour topic into more than one topic. */\nH5 { margin-top:3.00pt; margin-bottom:3.00pt; font-family:Verdana;\nfont-size:8pt; font-weight:bold; }\nH6 { margin-top:3.00pt; margin-bottom:3.00pt; font-family:Verdana;\nfont-size:8pt; font-weight:bold; }\n/* Use the Body style class for normal paragraphs. */\nP.Body { margin-top:6.00pt; margin-bottom:6.00pt; font-family:Verdana;\nfont-size:8pt; color:black; }\n/* Use the Anchor style class for graphic references on a line by themselves. */\nP.Anchor { margin-top:6.00pt; margin-bottom:6.00pt; font-family:Verdana;\nfont-size:10pt; color:black; }\n/* Use the Indent style classes to indent a paragraph. If you need to indent\ntext below a list item, use <br><br> to start the new paragraph within the same\nset of <li></li> tags. If you need to indent a list within another list, nest\nthe indented list within the first list's set of <ol></ol> or <ul></ul> tags. */\nP.Indent1 { margin-left:12.00pt; margin-top:6.00pt; margin-bottom:3.00pt;\nfont-family:Verdana; font-size:8pt; color:black; }\nP.Indent2 { margin-left:24.00pt; margin-top:6.00pt; margin-bottom:3.00pt;\nfont-family:Verdana; font-size:8pt; color:black; }\nP.Indent3 { margin-left:36.00pt; margin-top:6.00pt; margin-bottom:3.00pt;\nfont-family:Verdana; font-size:8pt; color:black; }\n/* Use the LI style for all list items. */\nLI { margin-top:3.00pt; margin-bottom:3.00pt; font-family:Verdana;\nfont-size:8pt; color:black; }\n/* Use the OL style for numbered lists. You do not have to type the number for\neach list item in a numbered list. */\nOL { margin-left:18.00pt; margin-top:3.00pt; margin-bottom:3.00pt;\ntext-indent:0pt; font-family:Verdana; font-size:8pt; color:black;\nlist-style-type: decimal; }\n/* Use the EquationNum style class for numbered lists of equations. You do not\nhave to type the number for each list item in a numbered list. */\nOL.EquationNum { margin-left:36.00pt; margin-top:3.00pt; margin-bottom:3.00pt;\ntext-indent:0pt; font-family:Verdana; font-size:8pt; color:black;\nlist-style-type: decimal; }\n/* Use the List-abc style class for lettered lists. You do not have to type the\nletter for each list item in a lettered list. */\nOL.List-abc { margin-left:18.00pt; margin-top:3.00pt; margin-bottom:3.00pt;\ntext-indent:0pt; font-family:Verdana; font-size:8pt; color:black;\nlist-style-type:lower-alpha; }\n/* Use the UL style for bulleted lists. You do not have to type the bullet for\neach list item in a bulleted list. */\nUL { margin-left:12.00pt; text-indent:0pt; margin-top:3.00pt;\nmargin-bottom:3.00pt; font-family:Verdana; font-size:8pt; color:black;\nlist-style-type: disc; }\n/* Use the List-Box style class for bulleted lists with boxes instead of\nbullets. You do not have to type the box for each list item in a box list. */\nUL.List-Box { margin-left:12.00pt; margin-top:3.00pt; margin-bottom:3.00pt;\ntext-indent:0pt; font-family:Verdana; font-size:8pt; color:black;\nlist-style-type: square; }\n/* Use the List-Diamond style class for bulleted lists with diamonds instead of\nbullets. You do not have to type the diamond for each list item in a diamond\nlist. */\nUL.List-Diamond { margin-left:12.00pt; margin-top:3.00pt; margin-bottom:3.00pt;\ntext-indent:0pt; font-family:Verdana; font-size:8pt; color:black;\nlist-style-image:url(diamond.gif); }\n/* Use the List-Hyphen style class for bulleted lists with hyphens instead of\nbullets. You do not have to type the hyphen for each list item in a hyphen list.\n*/\nUL.List-Hyphen { margin-left:12.00pt; margin-top:3.00pt; margin-bottom:3.00pt;\ntext-indent:0pt; font-family:Verdana; font-size:8pt; color:black;\nlist-style-image:url(hyphen.gif); }\n/* Use the Borderless style class for tables that do not need borders, such as\nfor 2-column or 3-column lists with no headings. */\nTable.Borderless { border:none; }\n/* Use the Bordered style class for tables that need borders. */\nTable.Bordered { border-width: 1pt; border-style: solid; border-color: black;\nborder-collapse: collapse; }\n/* Use the Borderless-Wide style class for tables that do not need borders and\nthat you want to stretch to fill the entire topic width. */\nTable.Borderless-Wide { border:none; width:100%; }\n/* Use the Bordered-Wide style class for tables that need borders and that you\nwant to stretch to fill the entire topic width. */\nTable.Bordered-Wide { border-width: 1pt; border-style: solid; border-color:\nblack; width:100%; border-collapse: collapse; }\n/* Use the TD style for table cells in Borderless or Borderless-Wide tables. */\nTD { font-family:Verdana; font-size:8pt; color:black; vertical-align:top;\npadding:3px; }\n/* Use the Bordered style class for table cells in Bordered or Bordered-Wide\ntables. */\nTD.Bordered { font-family:Verdana; font-size:8pt; color:black;\nvertical-align:top; border-width: 1pt; border-style: solid; border-color: black;\n}\n/* Use the Icon style class for table cells that contain note, caution, warning,\nor tip icons, or LabVIEW datatype terminals. */\nTD.Icon { width:40px; vertical-align:top; }\n/* Use the Table-cell-8pt style class for table cells in tables that contain a\nlot of information and need smaller text to fit it all on one screen to prevent\na horizontal scroll bar from appearing. */\nTD.Table-cell-8pt { font-family:Verdana; font-size:7pt; color:black; }\n/* Use the TH style for table heading cells in Borderless or Borderless-Wide\ntables. */\nTH { font-family:Verdana; font-size:8pt; color:black; font-weight:bold;\npadding:3px; }\n/* Use the Bordered style class for table heading cells in Bordered or\nBordered-Wide tables. */\nTH.Bordered { font-family:Verdana; font-size:8pt; color:black; font-weight:bold;\nborder-width: 1pt; border-style: solid; border-color: black; }\n/* Use the Table-cell-8pt style class for table heading cells in tables that\ncontain a lot of information and need smaller text to fit it all on one screen\nto prevent a horizontal scroll bar from appearing. */\nTH.Table-Head-8pt { font-family:Verdana; font-size:7pt; color:black;\nfont-weight:bold; }\n/* Use the Left-Align style class for table heading cells that you want to left\nalign instead of center align. */\nTH.Left-Align { font-family:Verdana; font-size:8pt; color:black;\nfont-weight:bold; padding:3px; text-align:left; }\n/***************************************************/\n/* CHARACTER FORMATS */\n/* The following section defines character formats that every HTML Help project\nshould need. */\n/* Use the Dark-Red format for warnings or cautions. */\n#Dark-Red { color: #800000 }\n/* Use the Monospace format for code or syntax examples. */\n#Monospace { font-family: Courier New; font-size: 8pt; }\n/* Use the Monospace-Bold format for messages and responses that the computer\nautomatically prints to the screen. */\n#Monospace-Bold { font-family: Courier New; font-size: 8pt; font-weight: bold; }\n/* Use the Monospace-Italic format to denote text that is a placeholder for a\nword or value that the user must supply. */\n#Monospace-Italic { font-family: Courier New; font-size: 8pt; font-style:\nitalic; }\n/* Use the Platform format to denote a specific platform. */\n#Platform { color: #0000FF; font-weight: bold; }\n/* Use the Symbol format for characters not in the Verdana character set. Use\nthis format sparingly. When possible, you should use the correct ASCII code for\nthe symbol or use a graphic to recreate the symbol. */\n#Symbol { font-family: Symbol; font-size: 8pt; }\n/* CHARACTER FORMATS Updated to conform with the CSE HTML Validator Pro */\n/* The following section defines character formats that every HTML Help project\nshould need. */\n/* Use the Dark-Red format for warnings or cautions. */\n.Dark-Red { color: #800000 }\n/* Use the Monospace format for code or syntax examples. */\n.Monospace { font-family: Courier New; font-size: 8pt; }\n/* Use the Monospace-Bold format for messages and responses that the computer\nautomatically prints to the screen. */\n.Monospace-Bold { font-family: Courier New; font-size: 8pt; font-weight: bold; }\n/* Use the Monospace-Italic format to denote text that is a placeholder for a\nword or value that the user must supply. */\n.Monospace-Italic { font-family: Courier New; font-size: 8pt; font-style:\nitalic; }\n/* Use the Platform format to denote a specific platform. */\n.Platform { color: #0000FF; font-weight: bold; }\n/* Use the Symbol format for characters not in the Verdana character set. Use\nthis format sparingly. When possible, you should use the correct ASCII code for\nthe symbol or use a graphic to recreate the symbol. */\n.Symbol { font-family: Symbol; font-size: 8pt; }\n/* Use the Red-text format to call attention to text that needs information\nadded or edited by techcomm */\n.Red-text {color: #FF0000;}\n/* Use the Green-Underline format for the green defintion in the conventions\ntopic */\n.Green-Underline {color: #007700; text-decoration : underline;}\n/* Use the glossButton format for the glossary buttons used in the glossary\ntopic */\n.glossButton { font-family:Verdana, sans-serif; font-size:12px; color:black; }\n/* Use for text sections and hyphenated words that should not break at line\nwraps */\nspan.nobreak{white-space:nowrap}\n/* The following styles define the color of links. */\na:link { color: #007700 }\na:hover { color: #FF0000 }\na:active { color: #FF0000 }\na:visited { color: #7F007F }\n/***************************************************/\n/* ACTIVITY STYLES */\n/* The following section defines styles that only tutorial-style HTML Help\nprojects should need. */\n/* Use the Activity-Objective style class for the objective at the beginning of\nan activity topic. */\nH3.Activity-Objective { color: #800000; }\n/***************************************************/\n/* CODE STYLES */\n/* The following section defines styles that you need to format entire sections\nof code or syntax examples. If you have just a few words you need to format as a\ncode or syntax example, use the Monospace character format. */\nP.Code { margin-top:3.00pt; margin-bottom:0.00pt; font-family:Courier New;\nfont-size:8pt; color:black; }\nP.Code1 { margin-left:12.00pt; margin-top:3.00pt; margin-bottom:0.00pt;\nfont-family:Courier New; font-size:8pt; color:black; }\nP.Code2 { margin-left:24.00pt; margin-top:3.00pt; margin-bottom:0.00pt;\nfont-family:Courier New; font-size:8pt; color:black; }\nP.Code3 { margin-left:36.00pt; margin-top:3.00pt; margin-bottom:0.00pt;\nfont-family:Courier New; font-size:8pt; color:black; }\n/***************************************************/\n/* FUNCTION STYLES */\n/* The following section defines styles that you might need to format function\nreference help. */\nP.F-VI-Code4 { margin-left:48.00pt; margin-top:3.00pt; margin-bottom:0.00pt;\nfont-family:Courier New; font-size:8pt; color:black; }\nP.F-VI-Code5 { margin-left:60.00pt; margin-top:3.00pt; margin-bottom:0.00pt;\nfont-family:Courier New; font-size:8pt; color:black; }\nP.F-VI-Equation { margin-top:9.00pt; margin-bottom:9.00pt; font-family:Verdana;\nfont-size:8pt; color:black; }\nOL.F-VI-EquationNum { margin-top:3.00pt; margin-bottom:3.00pt; text-indent:0pt;\nfont-family:Verdana; font-size:8pt; color:black; list-style-type: decimal; }\nCITE.expandspot { font-style : normal;\ncolor : green;\ncursor: hand;}\n.mvd-CITE-expandspot { font-style : normal;\ncolor : green;\ncursor: hand;}\nDFN.collapsed { font-style : italic;\nfont-weight : normal;\ndisplay : 'none';\ncolor : red;}\n.mvd-DFN-collapsed { font-style : italic;\nfont-weight : normal;\ndisplay : 'none';\ncolor : red;}\nDFN.expanded { font-style : italic;\nfont-weight : normal;\ncolor : red;}\n.mvd-DFN-expanded { font-style : italic;\nfont-weight : normal;\ncolor : red;}\nEM.dropspot { cursor : hand;\ncolor : green;}\n.mvd-EM-dropspot { cursor : hand;\ncolor : green;}\n</style>\n<noscript><p class=\"Body\"><strong>JavaScript\n(active content) is\ndisabled. For all content to be accessible, you must enable JavaScripts\nin your browser.</strong></p>\n</noscript>\n\n<body style=\"background-color: rgb(255, 255, 255);\">", "<h1>", "Product Full Name", w61, w59, " Readme</h1>\n<p class=\"Body\">" ("string"), "Month", w61, "Year", "</p>\n<p class=\"Body\">Thank you for using ", w60, ", version " ("string"), w59, ". The readme contains the following main sections:</p>\n<ul>" ("string"), w116, w113, w110, w108, w104, w102, w99, w96, w93, w89, w82, w81, w67, "</ul>\n" ("string")) -> (w79:string)
              n37 = Select(t=w71, s=w77, f="") -> (s? t:f=w70:string)
              n38 = Concatenate Strings(w79, w70) -> (w80:string)
            }
            frame "System Requirements" {
              n39 = Transpose 2D Array(2D array="SystemRequirements Table") -> (transposed array=w127:string[][])
              n40 = Index Array(array=w127) -> (element #1=w133:string[], element #2=w134:string[], element #3=w135:string[])  [unwired: 6 in]
              n41 = for {
                tunnel: w133 -> [w149] mode=indexing
                tunnel: w134 -> [w147] mode=indexing
                tunnel: w135 -> [w145] mode=indexing
                shift-right: [w150] -> w132
                shift-left: "" -> [w151]
                w146 = "<td class=\"Bordered\">\n" ("string")
                w144 = "\n</td>\n" ("string")
                n42 = Concatenate Strings(w151, "<tr>", w146, w149, w144, w146, w147, w144, w146, w145, w144) -> (w150:string)
              }
              n43 = Concatenate Strings("<h2><a name=\"sysRequire\"></a></h2>\n<h2>System\nRequirements</h2>\n<table class=\"Bordered\">\n<tbody>\n<tr>\n<th class=\"Bordered\">System Use</th>\n<th class=\"Bordered\">RAM</th>\n<th>Processor</th>\n</tr>" ("string"), w132, "</tbody>\n</table>\n" ("string")) -> (w138:string)
              n44 = local read "IsSysRequirements? chkBox"() -> (w140:bool)
              n45 = Select(t=w138, s=w140, f="") -> (s? t:f=w130:string)
              n46 = Concatenate Strings(w142, w130) -> (w141:string)
            }
            frame "Software Support" {
              n47 = call "_2D array to HTML.vi"("Table (2D Array)"="OperatingSystems Table") -> ("HTML Code"=w178:string)  [unwired: 14 in]
              n48 = Transpose 2D Array(2D array="NI Software Support Table") -> (transposed array=w159:string[][])
              n49 = Index Array(array=w159) -> (element #1=w158:string[], element #2=w157:string[])  [unwired: 4 in]
              n50 = for {
                shift-right: [w193] -> w156
                shift-left: "" -> [w194]
                tunnel: w158 -> [w191] mode=indexing
                tunnel: w157 -> [w189] mode=indexing
                n51 = Concatenate Strings(w194, "<tr align=\"center\">\n<td class=\"Bordered\" align=\"left\">" ("string"), w191, "</td>\n<td class=\"Bordered\">" ("string"), w189, "</td>\n</tr>\n" ("string")) -> (w193:string)
              }
              n52 = local read "IsSoftwareSupport? chkBox"() -> (w185:bool)
              n53 = Concatenate Strings("<p class=\"Body\"><strong>Note</strong>&nbsp;&nbsp;" ("string"), "OS Note", "</p>\n<p>\n<span class=\"Dark-Red\"><strong>Caution</strong>&nbsp;&nbsp;" ("string"), "Caution Text", "</span></p>\n" ("string"), "<p class=\"Body\">" ("string"), "Additional OS remarks", "</p>\n" ("string"), "<h3>NI Application Software Support </h3>\n<p class=\"Body\">The following table lists the NI\napplication software versions supported by " ("string"), w153, " " ("string"), w152, ".</p>\n<div class=\"DNL\">\n<table class=\"Bordered\">\n<tbody>\n<tr>\n<th class=\"Bordered\">NI Application Software</th>\n<th class=\"Bordered\">Supported Versions</th>\n</tr>\n" ("string"), w156, "</tbody>\n</table>\n</div>\n") -> (w154:string)
              n54 = Concatenate Strings("<a name=\"OS\"></a>\n<h2>Software Support in " ("string"), w153, "</h2>\n<h3>Operating System Support</h3>\n<p class=\"Body\">The following operating systems are\nsupported in " ("string"), w153, " " ("string"), w152, ": </p>\n<ul>\n" ("string"), w178, "\n</ul>\n" ("string"), w154) -> (w183:string)
              n55 = Select(t=w183, s=w185, f="") -> (s? t:f=w173:string)
              n56 = Concatenate Strings(w176, w173) -> (w175:string)
            }
            frame "Device Support" {
              n57 = call "_2D array to HTML.vi"("Table (2D Array)"="Device Support Table") -> ("HTML Code"=w196:string)  [unwired: 14 in]
              n58 = Concatenate Strings("<h2><a name=\"devSupport\"></a>Device Support in ", w195, "</h2>\n<p class=\"Body\">The following lists detail the devices\nsupported in " ("string"), w195, ".</p>\n<ul>" ("string"), w196, "</ul>\n" ("string")) -> (w200:string)
              n59 = local read "IsDeviceSupport? chkBox"() -> (w205:bool)
              n60 = Select(t=w200, s=w205, f="") -> (s? t:f=w202:string)
              n61 = Concatenate Strings(w207, w202) -> (w206:string)
            }
            frame "Upgrade Issues" {
              n62 = Concatenate Strings("<a name=\"upgrade\"></a>\n<h2>Upgrade and Compatibility Issues</h2>\n<p class=\"Body\">This section covers changes in" ("string"), w215, "functionality.</p>\n<h3>" ("string"), "Upgrade Issue Heading", "</h3>\n<p class=\"Body\">" ("string"), "UpgradeIssuesDescription", "</p>\n" ("string")) -> (w221:string)
              n63 = local read "IsUpgradeIssues? chkBox"() -> (w218:bool)
              n64 = Select(t=w221, s=w218, f="") -> (s? t:f=w222:string)
              n65 = Concatenate Strings(w219, w222) -> (w220:string)
            }
            frame "New Features" {
              w233 = " " ("string")
              n66 = call "_2D array to HTML.vi"("Table (2D Array)"="NewFeatures Table") -> ("HTML Code"=w227:string)  [unwired: 14 in]
              n67 = Concatenate Strings("<a name=\"New\"></a>\n<h2>New Features Added in " ("string"), w234, w233, w232, "</h2>\n<p class=\"Body\">The following features were added in" ("string"), w234, w233, w232, "</p>\n<ul>\n" ("string"), w227, "</ul>\n" ("string")) -> (w229:string)
              n68 = local read "IsNewFeatures? chkBox"() -> (w225:bool)
              n69 = Select(t=w229, s=w225, f="") -> (s? t:f=w239:string)
              n70 = Concatenate Strings(w237, w239) -> (w238:string)
            }
            frame "Fixed Issues" {
              n71 = Transpose 2D Array(2D array="FixedIssues Table") -> (transposed array=w247:string[][])
              n72 = Index Array(array=w247) -> (element #1=w246:string[], element #2=w245:string[])  [unwired: 4 in]
              n73 = for {
                shift-right: [w267] -> w243
                shift-left: "" -> [w268]
                tunnel: w246 -> [w265] mode=indexing
                tunnel: w245 -> [w263] mode=indexing
                n74 = Concatenate Strings(w268, "<tr class=\"DNL\">\n<td class=\"Bordered\">" ("string"), w265, "</td>\n<td class=\"Bordered\">" ("string"), w263, "</td>\n</tr>" ("string")) -> (w267:string)
              }
              n75 = Concatenate Strings("<a name=\"Fixed\"></a>\n<h2>Fixed Issues</h2>\n<p class=\"Body\">The following issues were fixed in" ("string"), w252, " " ("string"), w250, "</p>\n<div class=\"DNL\">\n<table class=\"Bordered\">\n<tbody>\n<tr>\n<th class=\"Bordered\">Issue ID</th>\n<th class=\"Bordered\">Summary</th>\n</tr>" ("string"), w243, "</tbody>\n</table>\n</div>" ("string")) -> (w258:string)
              n76 = local read "IsFixedIssues? chkBox"() -> (w255:bool)
              n77 = Select(t=w258, s=w255, f="") -> (s? t:f=w259:string)
              n78 = Concatenate Strings(w257, w259) -> (w256:string)
            }
            frame "Developer" {
              n79 = Concatenate Strings("<a name=\"Developer\"></a>\n<h2>Developer(s) of " ("string"), w276, "</h2>\n<p class=\"Body\">This application was developed by " ("string"), "AppDeveloper", "</p>\n<p class=\"Body\">Last upgrade of this application (to the version " ("string"), w272, ") was made by " ("string"), "AppUpgrader", "</p>\n" ("string")) -> (w277:string)
              n80 = local read "IsDeveloper? chkBox"() -> (w279:bool)
              n81 = Select(t=w277, s=w279, f="") -> (s? t:f=w283:string)
              n82 = Concatenate Strings(w282, w283) -> (w281:string)
            }
            frame "Contact Support" {
              n83 = Concatenate Strings("<a name=\"Support\"></a>\n<h2>Contact Support</h2>\n<p class=\"Body\">You can contact our support staff by one\nof the following:</p>\n<p class=\"Body\"><span style=\"font-weight: bold;\">Telephone:&nbsp;</span>" ("string"), "SupportTelephone", "</p>\n<p class=\"Body\"><span style=\"font-weight: bold;\">Email:&nbsp;</span>" ("string"), "SupportEmail", "</p>\n<p class=\"Body\"><span style=\"font-weight: bold;\">Community\nForums:&nbsp;</span>" ("string"), "Support CommunityForums", "</p>\n<hr>" ("string")) -> (w294:string)
              n84 = local read "IsContactSupport? chkBox"() -> (w286:bool)
              n85 = Select(t=w294, s=w286, f="") -> (s? t:f=w297:string)
              n86 = Concatenate Strings(w296, w297) -> (w295:string)
            }
            frame "Copyright" {
              n87 = Concatenate Strings("<a name=\"Copyright\"></a>\n<h3><strong>Copyright</strong></h3>\n<p class=\"Body\">" ("string"), "Copyright", "</p>\n" ("string")) -> (w305:string)
              n88 = local read "IsCopyright? chkBox"() -> (w301:bool)
              n89 = Select(t=w305, s=w301, f="") -> (s? t:f=w308:string)
              n90 = Concatenate Strings(w307, w308) -> (w306:string)
            }
            frame "Trademarks" {
              n91 = Concatenate Strings("<a name=\"Trademarks\"></a>\n<h3><strong>Trademarks</strong></h3>\n<p class=\"Body\">" ("string"), "Trademarks", "</p>\n" ("string")) -> (w316:string)
              n92 = local read "IsTrademarks? chkBox"() -> (w315:bool)
              n93 = Select(t=w316, s=w315, f="") -> (s? t:f=w319:string)
              n94 = Concatenate Strings(w318, w319) -> (w317:string)
            }
            frame "Patents" {
              n95 = Concatenate Strings("<a name=\"Patents\"></a>\n<h3><strong>Patents</strong></h3>\n<p class=\"Body\">" ("string"), "Patents", "</p>\n" ("string")) -> (w325:string)
              n96 = local read "IsPatents? chkBox"() -> (w327:bool)
              n97 = Select(t=w325, s=w327, f="") -> (s? t:f=w330:string)
              n98 = Concatenate Strings(w329, w330) -> (w328:string)
            }
            frame "Disclaimer" {
              n99 = Concatenate Strings("<a name=\"Patents\"></a>\n<h3><strong>Patents</strong></h3>\n<p class=\"Body\">" ("string"), "Disclaimer", "\n</p>" ("string")) -> (w337:string)
              n100 = local read "IsDisclaimer? chkBox"() -> (w341:bool)
              n101 = Select(t=w337, s=w341, f="") -> (s? t:f=w345:string)
              n102 = Concatenate Strings(w340, w345, "</body></html>" ("string")) -> (w343:string)
            }
            frame "Shutdown" {
            }
          }
        }
        n103 = Write to Text File(file (use dialog)=w47, text=w46) -> (refnum out=w44:refnum<file>, error out=w45:errorcluster)  [unwired: 2 in, 1 out]
        n104 = Close File(refnum=w44, error in=w45) -> (error out=→"error out":errorcluster)  [unwired: 1 out]
      }
      frame "Shutdown" {
      }
    }
  }
  "HTML File Path" <- w3
